vi "Test invalid table name.vi"(11 "Test Case In":refnum<class "Test Open Xml.lvclass">) -> (0 "error out":errorcluster, 3 "Test Case Out":refnum<class "Test Open Xml.lvclass">)   [LabVIEW 2020, in "Test Open Xml.lvclass"]
uses:
  Test Open Xml.lvclass
  C:/Program Files/National Instruments/LabVIEW 2025/vi.lib/Astemes/LUnit/Test Case.lvclass
  <vilib>/Astemes/LUnit/Test Case.lvclass/Test Case.ctl
  Test Open Xml.lvclass/Test Open Xml.ctl
  Source/Open Xml.lvlib
  <vilib>/Astemes/LUnit/Test Case.lvclass
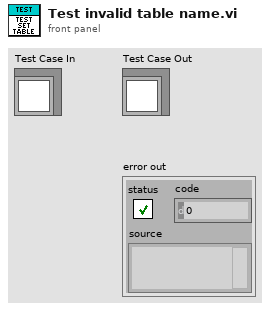
[diagram p1: front panel]
types:
  T1 = cluster{"Sheet Name":string, "Name":string, "Display Name":string, "Range":string}
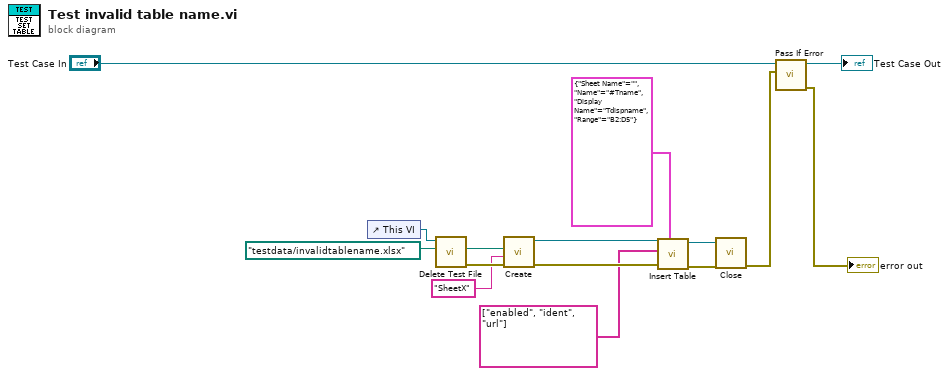
[diagram p0: block diagram]
diagram:
  n1 = control-ref of="This VI"() -> (w7:refnum<vi>)
  n2 = call "Delete Test File.vi"("name or relative path"=path "testdata/invalidtablename.xlsx", "VI in"=w7) -> ("error out"=w8:errorcluster, "deleted path"=w9:path)  [unwired: 8 in]
  n3 = call "Create.vi"("error in"=w8, "SheetName"="SheetX", "Path"=w9) -> ("error out"=w4:errorcluster, "SpreadsheetDoc"=w5:refnum<k24>)  [unwired: 7 in]
  n4 = call "Insert Table.vi"("Location"=T1 {"Sheet Name"="", "Name"="#Tname", "Display Name"="Tdispname", "Range"="B2:D5"}, "error in"=w4, "Header Names"=string[] ["enabled", "ident", "url"], "SpreadsheetDoc in"=w5) -> ("error out"=w12:errorcluster, "SpreadsheetDoc out"=w11:refnum<k24>)  [unwired: 6 in]
  n5 = call "Close.vi"("error in"=w12, "SpreadsheetDoc"=w11) -> ("error out"=w1:errorcluster)  [unwired: 9 in]
  n6 = call <vilib>:"Pass If Error.vi"("Assert error"=w1, "LUnit Test Case In"="Test Case In") -> ("error out"=→"error out":errorcluster, "LUnit Test Case Out"=→"Test Case Out":refnum<class "Test Open Xml.lvclass">)  [unwired: 8 in]
